vi "get handler reference.vi"(11 "Basic HTTP server.lvclass":refnum<class "Basic HTTP server.lvclass">) -> (3 "VI Name":string)   [LabVIEW 2016, in "Basic HTTP server.lvclass"]
uses:
  Basic HTTP server.lvclass
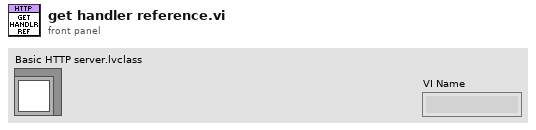
[diagram p1: front panel]
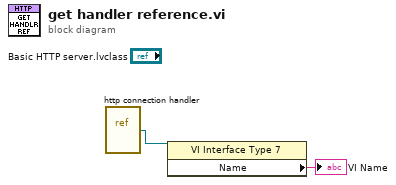
[diagram p0: block diagram]
diagram:
  n1 = vi-ref "http connection handler.vi"() -> (w2:refnum<vi>)
  n2 = property class="VI Interface Type 7"(reference=w2) -> ("Name"=→"VI Name":string)  [unwired: 1 in, 2 out]
